vi "Confirure FIFO Depths (SubVI).vi"(8 "error in (no error)":errorcluster, 11 "Refnum in":T1) -> (0 "error out":errorcluster, 1 "Actual Depth 3":u32, 2 "Actual Depth 2":u32, 3 "Refnum out":T1, 4 "Actual Depth 4":u32, 5 "Actual Depth 1":u32)   [LabVIEW 2017, in "SoC IP Library.lvlib"]
uses:
  SoC IP Library.lvlib
  Controls/FPGA Reference Type.ctl
  <vilib>/Utility/error.llb/Error Cluster From Error Code.vi
  <vilib>/rvi/interface/common/niFpgaWaitOnOcc.vi
  <vilib>/rvi/interface/nirviMethod/nirviMethod.xnode
  <vilib>/FPGAPlugInAG/Dynamic/niLvFpga_ConfigureFifo_Dynamic.vi
  <vilib>/rvi/errors/niLvFpgaMergeErrorWithErrorCode.vi
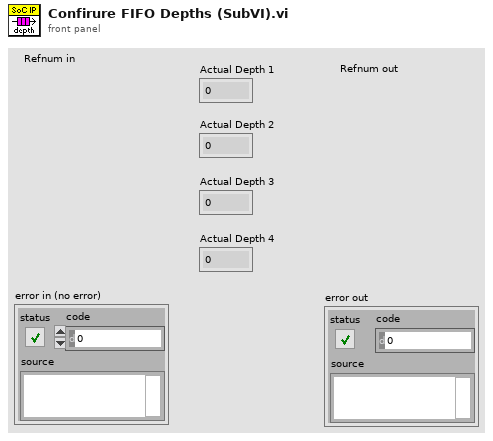
[diagram p1: front panel]
types:
  T1 = typedef "SoC IP Library.lvlib/FPGA Reference Type.ctl" = refnum<k20>
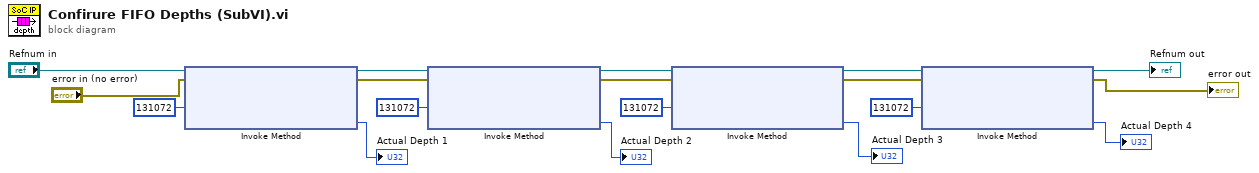
[diagram p0: block diagram]
diagram:
  n1 = xnode "Invoke Method"("FPGA VI Reference In"="Refnum in", "error in"="error in (no error)", "Requested Depth"=u32 131072) -> ("FPGA VI Reference Out"=w8:T1, "error out"=w11:errorcluster, "Actual Depth"=→"Actual Depth 1":u32)
  n2 = xnode "Invoke Method"("FPGA VI Reference In"=w8, "error in"=w11, "Requested Depth"=u32 131072) -> ("FPGA VI Reference Out"=w9:T1, "error out"=w12:errorcluster, "Actual Depth"=→"Actual Depth 2":u32)
  n3 = xnode "Invoke Method"("FPGA VI Reference In"=w9, "error in"=w12, "Requested Depth"=u32 131072) -> ("FPGA VI Reference Out"=w10:T1, "error out"=w13:errorcluster, "Actual Depth"=→"Actual Depth 3":u32)
  n4 = xnode "Invoke Method"("FPGA VI Reference In"=w10, "error in"=w13, "Requested Depth"=u32 131072) -> ("FPGA VI Reference Out"=→"Refnum out":T1, "error out"=→"error out":errorcluster, "Actual Depth"=→"Actual Depth 4":u32)
